vi "HovaCAL set Konzentrationen.vi"(8 "Fehler (Eingang, kein Fehler)":errorcluster, 11 "TestKonfig (Eingang)":T1 {"TestKonfig Interferent"."Gasflasche MFC3" items=["----"=10000, "IAG NH3 3000"=0, "IAG NH3 200"=1, "IAG NH3 2000"=2, "IAG MG"=3, "IAG O2"=4]; "TestKonfig Interferent"."Gasflasche MFC2" items=["----"=10000, "IAG NH3 3000"=0, "IAG NH3 200"=1, "IAG NH3 2000"=2, "IAG MG"=3, "IAG O2"=4]; "TestKonfig Interferent"."Eingangs Konzentration MFC1" min=0.0; "TestKonfig Interferent"."Ausgangs Konzentration MFC1" min=0.0; "TestKonfig Interferent"."MFC2" items=["MFC 2", "MFC 3", "MFC 4", "MFC 5"]; "TestKonfig Interferent"."MFC3" items=["MFC 2", "MFC 3", "MFC 4", "MFC 5"]; "TestKonfig Interferent"."Ausgangs Konzentration MFC3" min=0.0; "TestKonfig Interferent"."Eingangs Konzentration MFC3" min=0.0; "TestKonfig Interferent"."Ausgangs Konzentration MFC2" min=0.0; "TestKonfig Interferent"."Eingangs Konzentration MFC2" min=0.0; "TestKonfig H2O"."HovaCAL Temperature" format="%.2f"; "TestKonfig H2O"."HovaCAL Flow Input Cluster"."HovaCAL Flow Input Cluster" format="%.2f"; "TestKonfig H2O"."Eingangs Konzentration:" min=0.0; "TestKonfig H2O"."zusätzliche Zeitdauer Erster Punkt" min=30 step=1 format="%#_5g"; "TestKonfig H2O"."Zeitdauer Stufen" format="%#_5g"; "TestKonfig H2O"."Max Fehler" format="%#_5g"; "TestKonfig H2O"."Anzahl Stufen" format="%#_5g"; "TestKonfig H2O"."Modus" items=["Messen", "CG zu Entnahmestelle"]}) -> (0 "Fehler (Ausgang)":errorcluster)   [LabVIEW 2020, in "EPA 1065.lvlib" / "HovaCAL Interference verificaton.lvlib"]
uses:
  HovaCAL Interference verificaton.lvlib
  TestKonfig.ctl
  TestKonfig H2O.ctl
  Modus.ctl
  Linearisierung V2/SpanEinstellungen/Einheit.ctl
  Linearisierung V2/Gasteiler/Stufen Tabelle.ctl
  Linearisierung V2/Gasteiler/HovaCAL_Interface/Controls/Flow Einstellung.ctl
  Linearisierung V2/Gasteiler/HovaCAL_Interface/Controls/Temp Sollwerte Anzeige.ctl
  TestKonfig Interferents.ctl
  MFCAuswahl.ctl
  Seiten/System Einstellungen V2/Gasflasche Auswahl.ctl
  Linearisierung V2/Gasteiler/HovaCAL_Interface/Kommunikation/Aktion_FGV_HovaCAL_Interface_SetData.ctl
  Linearisierung V2/Gasteiler/HovaCAL_Interface/Kommunikation/Kommunikation.lvlib
  Linearisierung V2/SpanEinstellungen/SpanEinstellungen.lvlib
  Linearisierung V2/Gasteiler/Gasteiler.lvlib
  Linearisierung V2/Gasteiler/HovaCAL_Interface/Controls/Controls.lvlib
  Seiten/System Einstellungen V2/System Einstellungen V2.lvlib
panel:
  # "sec"
  # "%"
  # "sec"
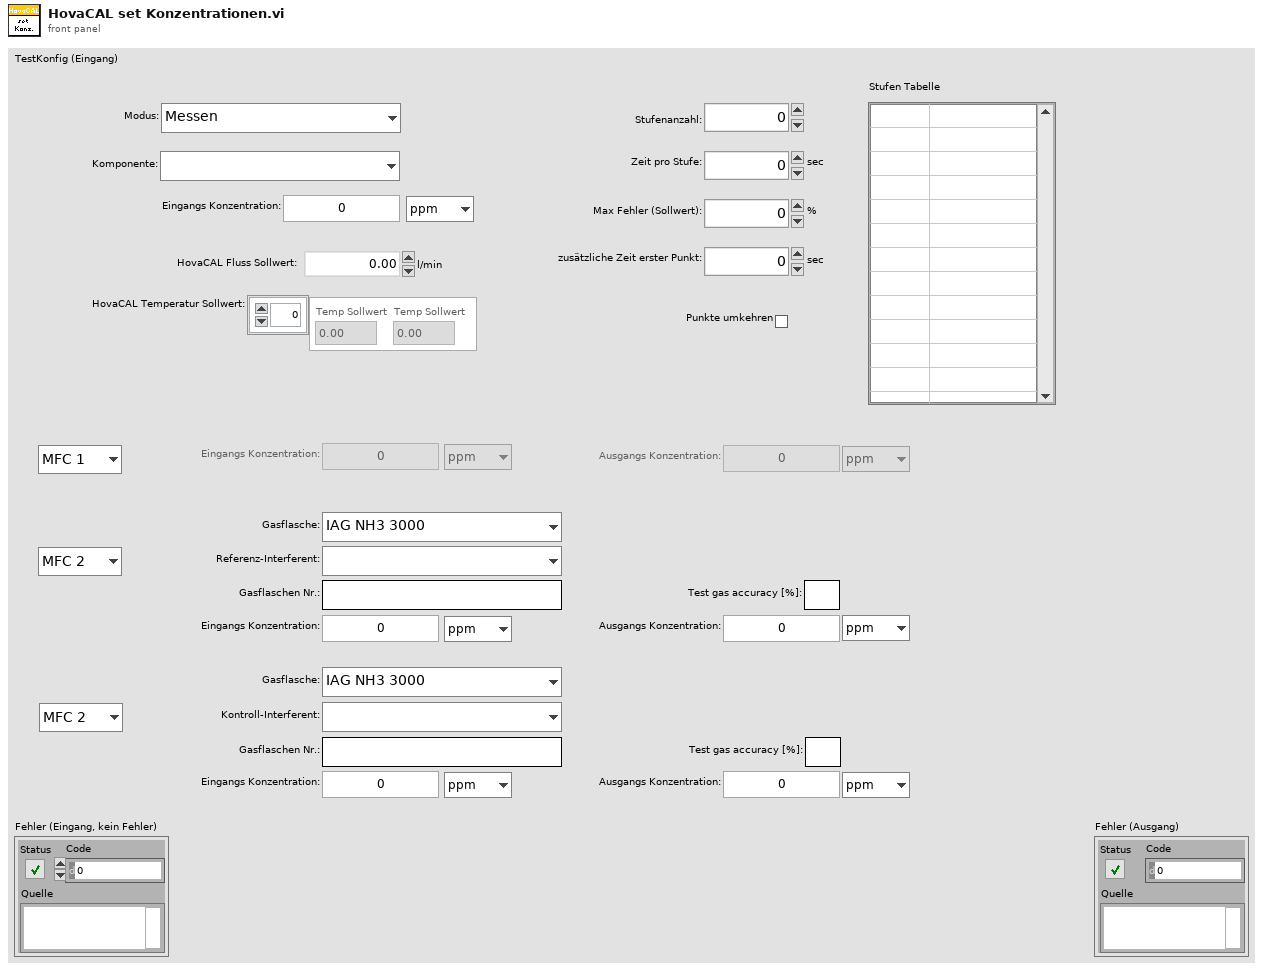
[diagram p1: front panel]
types:
  T1 = typedef "EPA 1065.lvlib/HovaCAL Interference verificaton.lvlib/TestKonfig.ctl" = cluster{"TestKonfig H2O":T2, "TestKonfig Interferent":T8}
  T2 = typedef "EPA 1065.lvlib/HovaCAL Interference verificaton.lvlib/TestKonfig H2O.ctl" = cluster{"Modus":T3, "Komponente:":u16, "Eingangs Konzentration:":dbl, "Einheit":T4, "Anzahl Stufen":sgl, "Zeitdauer Stufen":sgl, "Max Fehler":sgl, "zusätzliche Zeitdauer Erster Punkt":sgl, "Punkte umkehren":bool, "Stufen Tabelle":T5, "HovaCAL Flow Input Cluster":T6, "HovaCAL Temperature":T7}
  T3 = typedef "EPA 1065.lvlib/HovaCAL Interference verificaton.lvlib/Modus.ctl" = u16
  T4 = typedef "Linearisierung v2.lvlib/SpanEinstellungen.lvlib/Einheit.ctl" = enum16{"ppm", "%"}
  T5 = typedef "Linearisierung v2.lvlib/Gasteiler.lvlib/Stufen Tabelle.ctl" = string[][]
  T6 = typedef "Linearisierung v2.lvlib/Gasteiler.lvlib/HovaCAL_Interface.lvlib/Controls.lvlib/Flow Einstellung.ctl" = cluster{"HovaCAL Flow Input Cluster":dbl}
  T7 = typedef "Linearisierung v2.lvlib/Gasteiler.lvlib/HovaCAL_Interface.lvlib/Controls.lvlib/Temp Sollwerte Anzeige.ctl" = dbl[]
  T8 = typedef "EPA 1065.lvlib/HovaCAL Interference verificaton.lvlib/TestKonfig Interferents.ctl" = cluster{"MFC1":enum16{"MFC 1"}, "Eingangs Konzentration MFC1":dbl, "Einheit MFC1 Eingang":T4, "Ausgangs Konzentration MFC1":dbl, "Einheit MFC1 Ausgang":T4, "MFC2":T9, "Referenz-Interferent:":u16, "Gasflaschen Nr MFC2":string, "Accuracy MFC2":string, "Eingangs Konzentration MFC2":dbl, "Einheit MFC2 Eingang":T4, "Ausgangs Konzentration MFC2":dbl, "Einheit MFC2 Ausgang":T4, "MFC3":T9, "Kontroll-Interferent:":u16, "Gasflaschen Nr MFC3":string, "Accuracy MFC3":string, "Eingangs Konzentration MFC3":dbl, "Einheit MFC3 Eingang":T4, "Ausgangs Konzentration MFC3":dbl, "Einheit MFC3 Ausgang":T4, "Gasflasche MFC2":T10, "Gasflasche MFC3":T10}
  T9 = typedef "EPA 1065.lvlib/HovaCAL Interference verificaton.lvlib/MFCAuswahl.ctl" = u16
  T10 = typedef "System Einstellungen V2.lvlib/Gasflasche Auswahl.ctl" = u16
  T11 = cluster{"input concentration setpoint":dbl, "output concentration setpoint":dbl}
  T12 = typedef "Linearisierung v2.lvlib/Gasteiler.lvlib/HovaCAL_Interface.lvlib/Kommunikation.lvlib/Aktion_FGV_HovaCAL_Interface_SetData.ctl" = enum16{"lesen", "Konzentrationen", "Pumpen Parameter", "Pumpe Konzentration", "Pumpe run", "Temperaturen", "Fluss", "Limits", "init"}
  T13 = cluster{"input concentration setpoint":dbl, "output concentration setpoint":dbl}[]
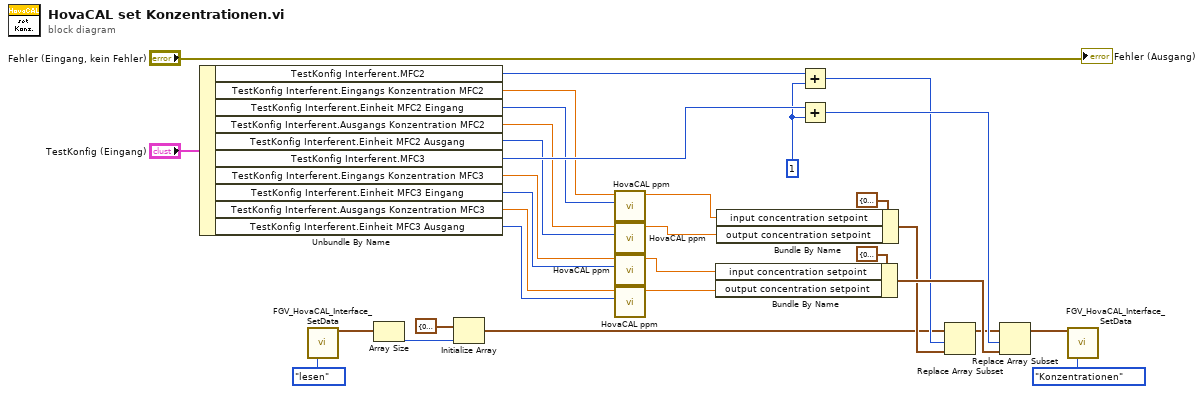
[diagram p0: block diagram]
diagram:
  w19 = u16 1 ("x+y")
  n1 = Unbundle By Name("TestKonfig (Eingang)") -> ("TestKonfig Interferent.MFC2"=w20:T9, "TestKonfig Interferent.Eingangs Konzentration MFC2"=w11:dbl, "TestKonfig Interferent.Einheit MFC2 Eingang"=w12:T4, "TestKonfig Interferent.Ausgangs Konzentration MFC2"=w9:dbl, "TestKonfig Interferent.Einheit MFC2 Ausgang"=w8:T4, "TestKonfig Interferent.MFC3"=w21:T9, "TestKonfig Interferent.Eingangs Konzentration MFC3"=w6:dbl, "TestKonfig Interferent.Einheit MFC3 Eingang"=w5:T4, "TestKonfig Interferent.Ausgangs Konzentration MFC3"=w3:dbl, "TestKonfig Interferent.Einheit MFC3 Ausgang"=w1:T4)
  n2 = call "FGV_HovaCAL_Interface_SetData.vi"("Aktion"=Aktion_FGV_HovaCAL_Interface_SetData."lesen") -> ("Set Values Cluster out"=w22:T13)  [unwired: 8 in, 6 out]
  n3 = Array Size(array=w22) -> (size(s)=w17:i32)
  n4 = Initialize Array(T11 {"input concentration setpoint"=0.0, "output concentration setpoint"=0.0} ("Set Values Cluster out"), w17) -> (w13:T13)
  n5 = call "HovaCAL ppm.vi"("Einheit MFC2 Eingang"=w12, "Eingangs Konzentration MFC2"=w11) -> ("Numerisch"=w10:dbl)  [unwired: 9 in]
  n6 = call "HovaCAL ppm.vi"("Einheit MFC2 Eingang"=w8, "Eingangs Konzentration MFC2"=w9) -> ("Numerisch"=w7:dbl)  [unwired: 9 in]
  n7 = call "HovaCAL ppm.vi"("Einheit MFC2 Eingang"=w5, "Eingangs Konzentration MFC2"=w6) -> ("Numerisch"=w4:dbl)  [unwired: 9 in]
  n8 = call "HovaCAL ppm.vi"("Einheit MFC2 Eingang"=w1, "Eingangs Konzentration MFC2"=w3) -> ("Numerisch"=w2:dbl)  [unwired: 9 in]
  n9 = Bundle By Name(cluster=T11 {"input concentration setpoint"=0.0, "output concentration setpoint"=0.0} ("Set Values Cluster out"), "input concentration setpoint"=w4, "output concentration setpoint"=w2) -> (w29:T11)
  n10 = Bundle By Name(cluster=T11 {"input concentration setpoint"=0.0, "output concentration setpoint"=0.0} ("Set Values Cluster out"), "input concentration setpoint"=w10, "output concentration setpoint"=w7) -> (w27:T11)
  n11 = Add(x=w20, y=w19) -> (x+y=w23:T9)
  n12 = Add(x=w21, y=w19) -> (x+y=w25:T9)
  n13 = Replace Array Subset(array=w13, new element=w27, index=w23) -> (w24:T13)
  n14 = Replace Array Subset(array=w24, new element=w29, index=w25) -> (w30:T13)
  n15 = call "FGV_HovaCAL_Interface_SetData.vi"("Set Values Cluster in"=w30, "Aktion"=Aktion_FGV_HovaCAL_Interface_SetData."Konzentrationen") -> ()  [unwired: 7 in, 7 out]
  "Fehler (Ausgang)" <- "Fehler (Eingang, kein Fehler)"
